vi "Resource Editor.vi"(7 "Load from Initial Path (F)":bool, 10 "Initial Resources":T1, 11 "Path":path) -> (2 "Final Resources":T1)   [LabVIEW 2018]
doc: "Edits several types of LabVIEW files at a low level, including VI's.\n\nCan also be used as a dialog subVI for editing resource clusters."
uses:
  Resource Array.ctl
  Resource.ctl
  Resource Editor Internal Commands Enum.ctl
panel:
  in  "Delete":bool
  in  "Add":bool
  in  "Name":string
  in  "Type":string
  in  "ID":i32
  in  "Export":bool
  in  "Import":bool
  in  "Paste":bool
  in  "Copy":bool
  in  "XML":bool
  in  "Fix MD5":bool
  in  "File type":string
  in  "Data":string
  in  "Hex view":bool
  in  "Save":bool
  in  "Load":bool
  in  "Resources":i32(listbox)
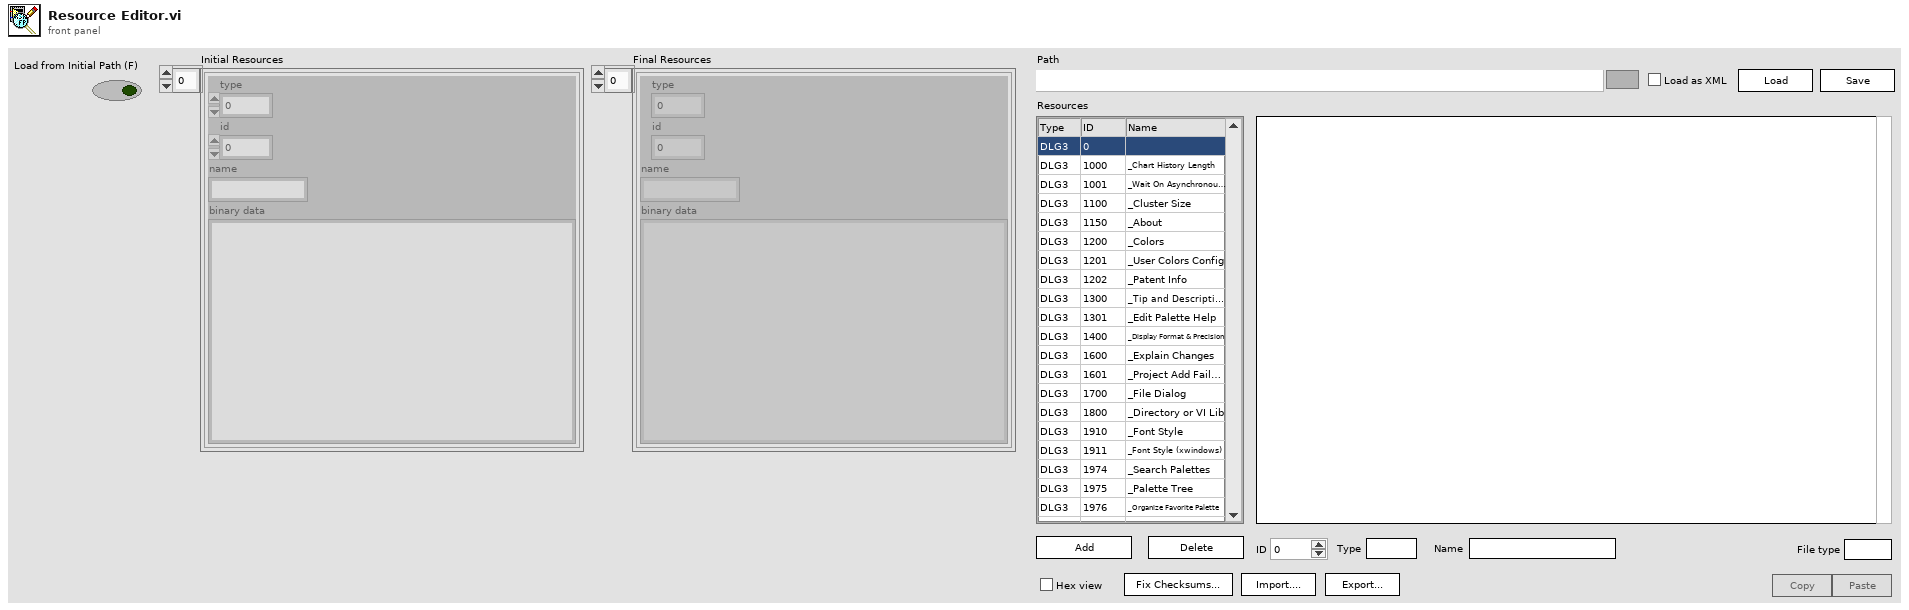
[diagram p1: front panel]
types:
  T1 = typedef "Resource Array.ctl" = T2[]
  T2 = typedef "Resource.ctl" = cluster{"type":u32, "id":i32, "name":string, "binary data":string}
  T3 = typedef "Resource Editor Internal Commands Enum.ctl" = enum16{"Refresh Resource List", "Load from Path"}
  T4 = enum8{"Enabled", "Disabled", "Disabled and Grayed Out"}
  T5 = enum16{"Left Button", "Center Button", "Right Button", "Window Close"}
  T6 = enum16{"open", "replace", "create", "open or create", "replace or create", "replace or create with confirmation"}
  T7 = cluster{"Numbers":u32, "Strings":u32, "Paths":u32}
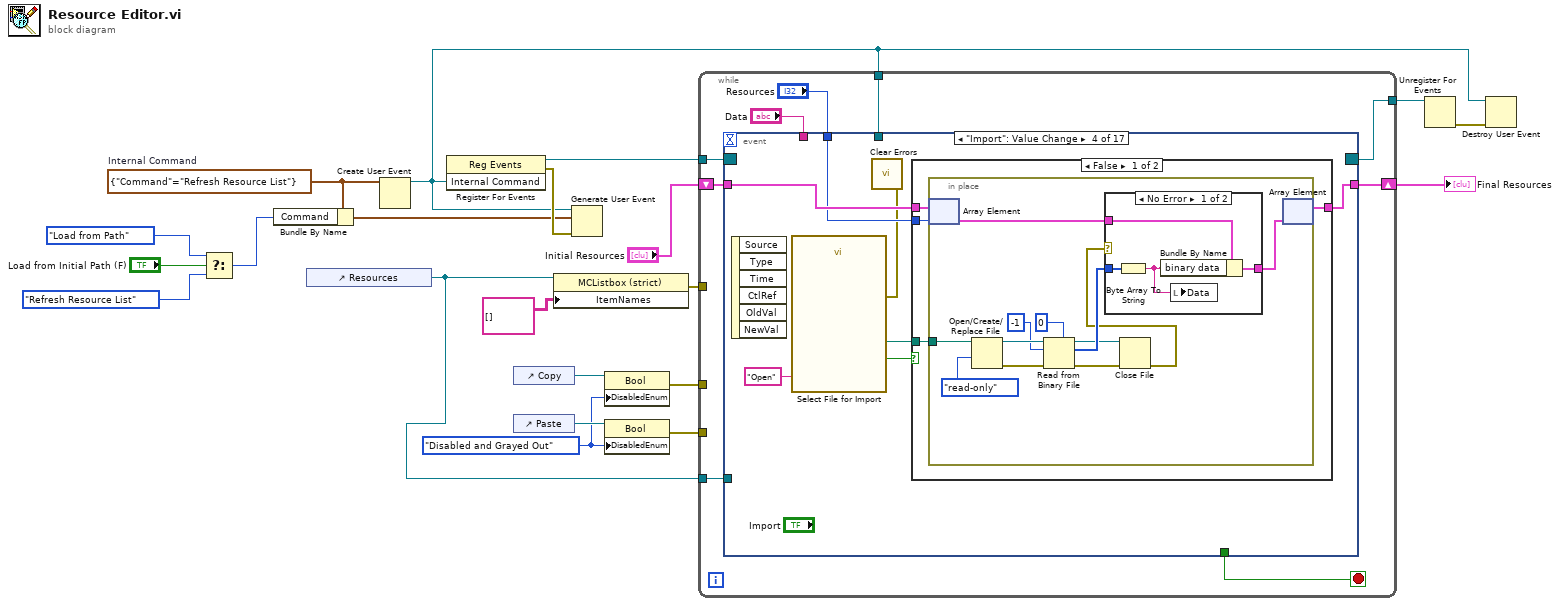
[diagram p0: block diagram]
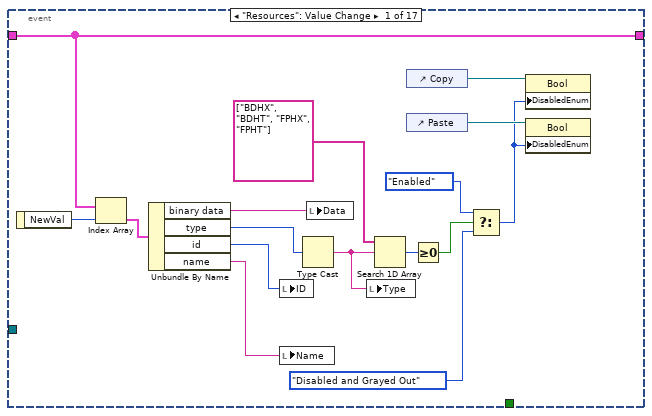
[diagram p2: hidden frame]
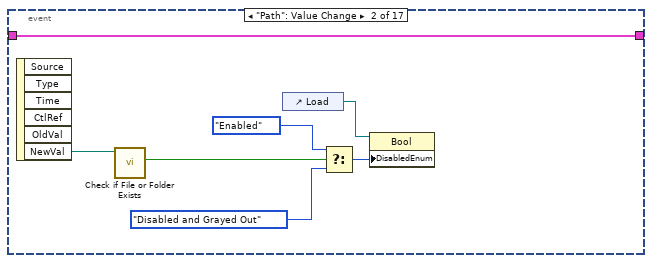
[diagram p3: hidden frame]
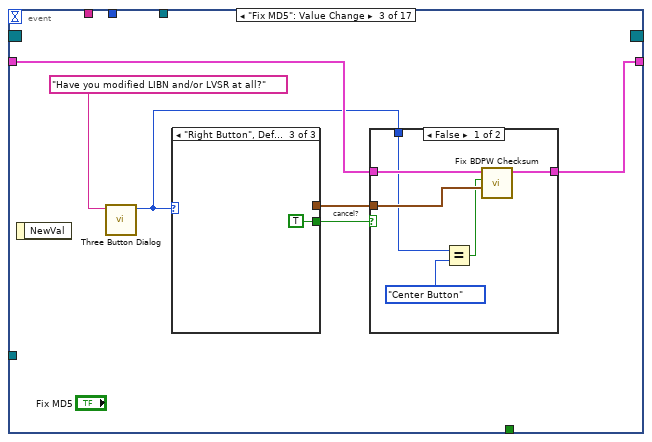
[diagram p4: hidden frame]
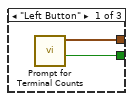
[diagram p5: hidden frame]
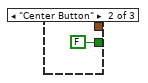
[diagram p6: hidden frame]
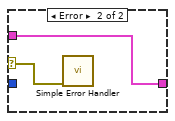
[diagram p8: hidden frame]
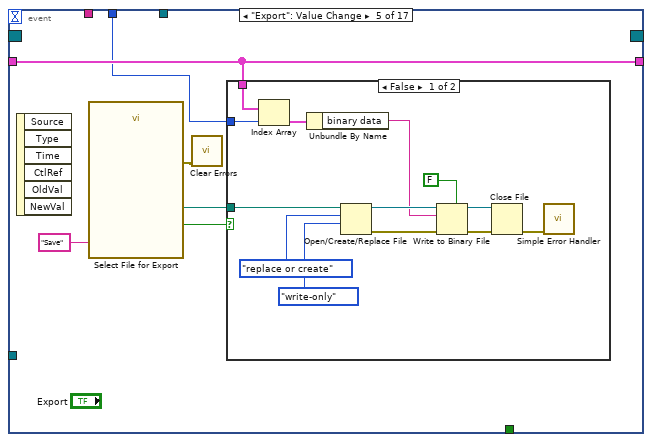
[diagram p10: hidden frame]
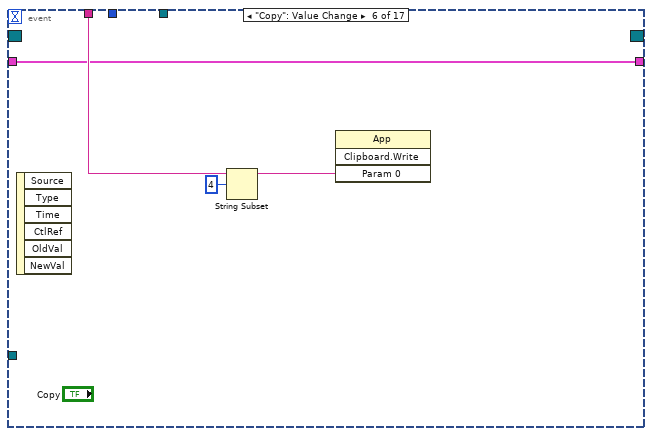
[diagram p12: hidden frame]
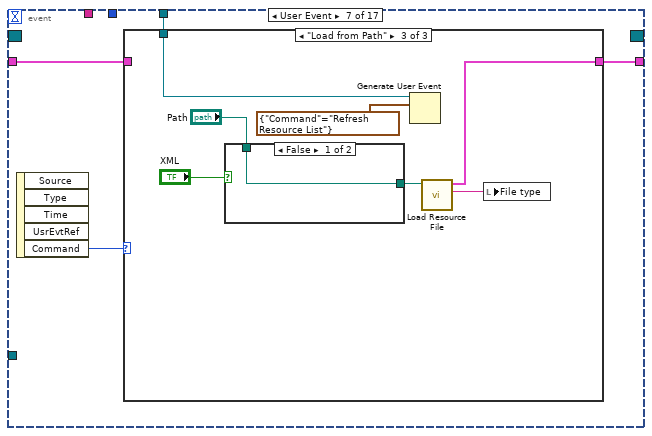
[diagram p13: hidden frame]
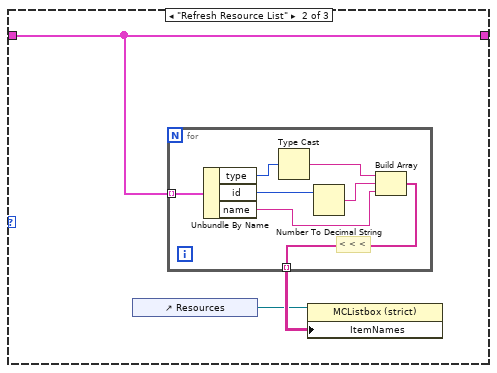
[diagram p15: hidden frame]
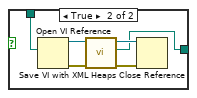
[diagram p16: hidden frame]
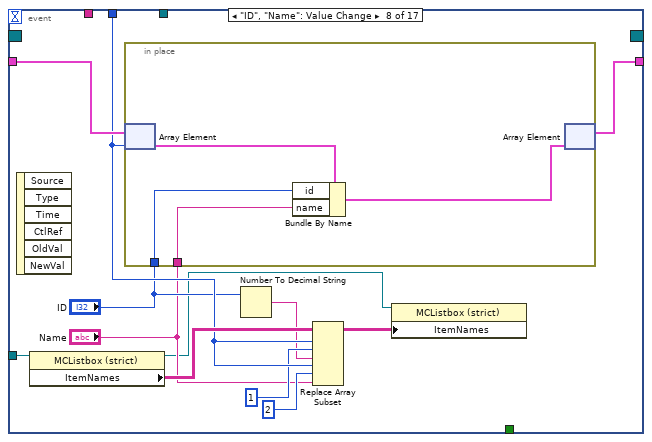
[diagram p17: hidden frame]
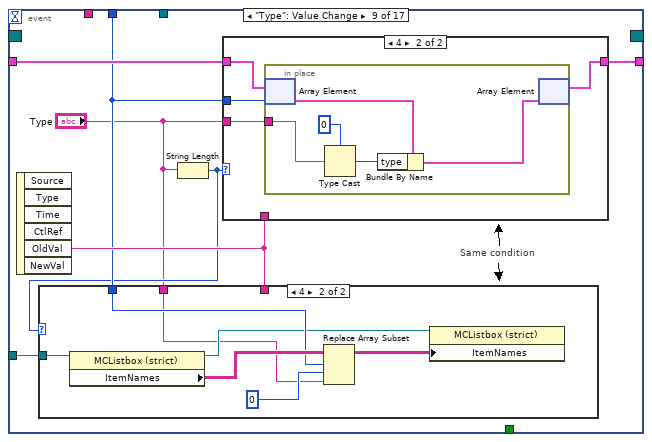
[diagram p18: hidden frame]
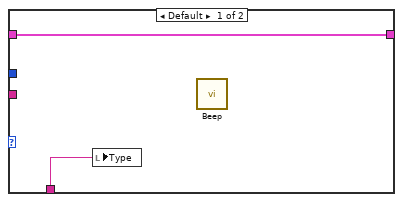
[diagram p20: hidden frame]
diagram:
  w6 = cluster{"Command":T3} {"Command"=enum."Refresh Resource List"}  # Internal Command
  w16 = T4."Disabled and Grayed Out" ("Disabled")
  n1 = Select(t=Resource_Editor_Internal_Commands_Enum."Load from Path" ("Command"), s="Load from Initial Path (F)", f=Resource_Editor_Internal_Commands_Enum."Refresh Resource List" ("Command")) -> (s? t:f=w1:T3)
  n2 = Bundle By Name(cluster=w6, "Command"=w1) -> (w5:cluster{"Command":T3})
  n3 = control-ref of="Resources"() -> (w13:refnum<vi>)
  n4 = Create User Event(user event datatype=w6) -> (user event=w7:refnum<user-event>)  [unwired: 1 in, 1 out]
  n5 = register-events(w7) -> (reference out=w8:refnum<event-registration>, error out=w9:errorcluster)  [unwired: 2 in]
  n6 = control-ref of="Copy"() -> (w18:refnum<vi>)
  n7 = control-ref of="Paste"() -> (w17:refnum<vi>)
  n8 = property class="MCListbox (strict)"(reference=w13, "ItemNames"=string[][] [] ("Item Names")) -> (error out=w20:errorcluster)  [unwired: 1 in, 1 out]
  n9 = Generate User Event(user event=w7, event data cluster=w5, error in=w9) -> ()  [unwired: 1 in, 2 out]
  n10 = property class="Bool"(reference=w18, "DisabledEnum"=w16) -> (error out=w15:errorcluster)  [unwired: 1 in, 1 out]
  n11 = property class="Bool"(reference=w17, "DisabledEnum"=w16) -> (error out=w14:errorcluster)  [unwired: 1 in, 1 out]
  n12 = while {
    shift-right: [w29] -> w12
    shift-left: "Initial Resources" -> [w30]
    tunnel: w20 -> [_]
    tunnel: w15 -> [_]
    tunnel: w14 -> [_]
    tunnel: w13 -> [w25]
    tunnel: w8 -> [w24]
    tunnel: w7 -> [w23]
    tunnel: [w22] -> w11
    stop <- w28 stop-if-true
    n13 = event shown="[3] \"Import\": Value Change" {
      selector: w24 -> [_ _ _ _ _ _ _ _ _ _ _ _ _ _ _ _ _]
      dyn-events: [_ _ _ _ _ _ _ _ _ _ _ _ _ _ _ _ _] -> w22
      timeout: _ -> [_ _ _ _ _ _ _ _ _ _ _ _ _ _ _ _ _]
      tunnel: w30 -> [w44 w47 w56 w77 w106 w122 w125 w164 w175 w202 w218 w227 w232 w239 w246 w251 w260]
      tunnel: [w44 w47 w59 w75 w106 w122 w126 w163 w174 w200 w216 w227 w232 w237 w244 w251 w260] -> w29
      tunnel: [_ _ _ _ _ _ _ _ _ _ _ _ _ _ _ _ w261] -> w28
      tunnel: "Data" -> [_ _ _ _ _ w123 _ _ _ _ _ _ _ _ _ _ _]
      tunnel: "Resources" -> [_ _ _ w76 w103 _ _ w161 w171 w201 w215 _ _ w233 w245 _ _]
      tunnel: w25 -> [_ _ _ _ _ _ _ w154 w173 _ _ _ _ _ _ _ _]
      tunnel: w23 -> [_ _ _ _ _ _ w124 _ _ _ _ _ w230 _ w243 _ _]
      event "Resources": Value Change {
        n14 = event-data() -> ("NewVal"=w46:i32)  [unwired: 1 in]
        n15 = Index Array(array=w44, index=w46) -> (element=w45:T2)
        n16 = Unbundle By Name(w45) -> ("binary data"=w43:string, "type"=w42:u32, "id"=w33:i32, "name"=w32:string)
        n17 = local write "ID"(w33) -> ()
        n18 = local write "Name"(w32) -> ()
        n19 = Type Cast(x=w42) -> (*(type *) &x=w31:string)  [unwired: 1 in]
        n20 = local write "Data"(w43) -> ()
        n21 = local write "Type"(w31) -> ()
        n22 = Search 1D Array(1D array=string[] ["BDHX", "BDHT", "FPHX", "FPHT"], element=w31) -> (index of element=w38:i32)  [unwired: 1 in]
        n23 = control-ref of="Copy"() -> (w40:refnum<vi>)
        n24 = control-ref of="Paste"() -> (w39:refnum<vi>)
        n25 = Greater Or Equal To 0?(x=w38) -> (x >= 0?=w37:bool)
        n26 = Select(t=T4."Enabled" ("Disabled"), s=w37, f=T4."Disabled and Grayed Out" ("Disabled")) -> (s? t:f=w34:T4)
        n27 = property class="Bool"(reference=w40, "DisabledEnum"=w34) -> ()  [unwired: 1 in, 2 out]
        n28 = property class="Bool"(reference=w39, "DisabledEnum"=w34) -> ()  [unwired: 1 in, 2 out]
      }
      event "Path": Value Change {
        n29 = event-data() -> ("NewVal"=w53:path)  [unwired: 1 in, 5 out]
        n30 = call <vilib>:"Check if File or Folder Exists.vi"("path"=w53) -> ("file or folder exists?"=w48:bool)  [unwired: 8 in, 2 out]
        n31 = control-ref of="Load"() -> (w52:refnum<vi>)
        n32 = Select(t=T4."Enabled" ("Disabled"), s=w48, f=T4."Disabled and Grayed Out" ("Disabled")) -> (s? t:f=w49:T4)
        n33 = property class="Bool"(reference=w52, "DisabledEnum"=w49) -> ()  [unwired: 1 in, 2 out]
      }
      event "Fix MD5": Value Change {
        # "cancel?"
        n34 = event-data() -> ()  [unwired: 1 in, 1 out]
        n35 = call <vilib>:"Three Button Dialog.vi"("message"="Have you modified LIBN and/or LVSR at all?") -> ("Which Button?"=w54:T5)  [unwired: 10 in]
        n36 = case shown="\"Right Button\", Default" w54 {
          tunnel: [w61 FALSE ("Canceled?") TRUE ("Canceled?")] -> w58
          tunnel: [w60 _ _] -> w57
          frame "Left Button" {
            n37 = call "Prompt for Terminal Counts.vi"() -> ("Canceled?"=w61:bool, "Terminal Counts"=w60:T7)  [unwired: 10 in]
          }
          frame "Center Button" {
          }
          frame "Right Button", Default {
          }
        }
        n38 = case shown="False" w58 {
          tunnel: w56 -> [w69 w70]
          tunnel: [w68 w70] -> w59
          tunnel: w57 -> [w67 _]
          tunnel: w54 -> [w65 _]
          frame False {
            n39 = Equal?(x=w65, y=T5."Center Button" ("Which Button?")) -> (x = y?=w64:bool)
            n40 = call "Fix BDPW Checksum.vi"("Terminal Counts"=w67, "Only fix 3rd hash (F)"=w64, "Resources in"=w69) -> ("Resources out"=w68:T1)  [unwired: 8 in]
          }
          frame True {
          }
        }
      }
      event "Import": Value Change {
        n41 = event-data() -> ()  [unwired: 1 in, 6 out]
        n42 = call "Select File for Import"("button label"="Open") -> ("selected path"=w73:path, "cancelled"=w74:bool, "error out"=w71:errorcluster)  [unwired: 11 in, 1 out]
        n43 = call <vilib>:"Clear Errors.vi"("error in (no error)"=w71) -> ()  [unwired: 5 in, 2 out]
        n44 = case shown="False" w74 {
          tunnel: w77 -> [w81 w100]
          tunnel: w76 -> [w80 _]
          tunnel: [w79 w100] -> w75
          tunnel: w73 -> [w78 _]
          frame False {
            n45 = in-place {
              in-place-border: w78 -> [w93]
              n46 = in-place-array #1(w81, w80) -> (w87:T2)
              n47 = Open/Create/Replace File(file path (use dialog)=w93, access (0:read/write)=enum16{"read/write", "read-only", "write-only"}."read-only") -> (refnum out=w91:refnum<file>, error out=w88:errorcluster)  [unwired: 4 in, 1 out]
              n48 = Read from Binary File(5:u8 0, 8:w88, 10:-1 ("count (1)"), 11:w91) -> (0:w83:errorcluster, 2:w86:u8[], 3:w84:refnum<file>)  [unwired: 2 in, 1 out]
              n49 = Close File(refnum=w84, error in=w83) -> (error out=w82:errorcluster)  [unwired: 1 out]
              n50 = case shown="No Error" w82 {
                selector: w82 -> [_ w98]
                tunnel: w87 -> [w97 w99]
                tunnel: w86 -> [w96 _]
                tunnel: [w95 w99] -> w85
                frame No Error {
                  n51 = Byte Array To String(unsigned byte array=w96) -> (string=w94:string)
                  n52 = Bundle By Name(cluster=w97, "binary data"=w94) -> (w95:T2)
                  n53 = local write "Data"(w94) -> ()
                }
                frame Error {
                  n54 = call <vilib>:"Simple Error Handler.vi"("error in (no error)"=w98) -> ()  [unwired: 4 in, 5 out]
                }
              }
              n55 = in-place-array #1(w85) -> (w79:T1)  [unwired: 1 out]
            }
          }
          frame True {
          }
        }
      }
      event "Export": Value Change {
        n56 = event-data() -> ()  [unwired: 1 in, 6 out]
        n57 = call "Select File for Export"("button label"="Save") -> ("selected path"=w104:path, "cancelled"=w105:bool, "error out"=w101:errorcluster)  [unwired: 11 in, 1 out]
        n58 = call <vilib>:"Clear Errors.vi"("error in (no error)"=w101) -> ()  [unwired: 5 in, 2 out]
        n59 = case shown="False" w105 {
          tunnel: w106 -> [w114 _]
          tunnel: w104 -> [w119 _]
          tunnel: w103 -> [w113 _]
          frame False {
            n60 = Index Array(array=w114, index=w113) -> (element=w112:T2)
            n61 = Unbundle By Name(w112) -> ("binary data"=w111:string)
            n62 = Open/Create/Replace File(file path (use dialog)=w119, operation (0:open)=T6."replace or create", access (0:read/write)=enum16{"read/write", "read-only", "write-only"}."write-only") -> (refnum out=w115:refnum<file>, error out=w108:errorcluster)  [unwired: 3 in, 1 out]
            n63 = Write to Binary File(file (use dialog)=w115, data=w111, error in=w108, 5:FALSE ("prepend array or string size? (T)")) -> (refnum out=w109:refnum<file>, error out=w110:errorcluster)  [unwired: 2 in, 1 out]
            n64 = Close File(refnum=w109, error in=w110) -> (error out=w107:errorcluster)  [unwired: 1 out]
            n65 = call <vilib>:"Simple Error Handler.vi"("error in (no error)"=w107) -> ()  [unwired: 4 in, 5 out]
          }
          frame True {
          }
        }
      }
      event "Copy": Value Change {
        n66 = event-data() -> ()  [unwired: 1 in, 6 out]
        n67 = String Subset(string=w123, offset (0)=4) -> (substring=w121:string)  [unwired: 1 in]
        n68 = invoke class="App" method="Clipboard.Write"("Param 0"=w121) -> ()  [unwired: 3 in, 4 out]
      }
      event User Event {
        n69 = event-data() -> ("Command"=w127:T3)  [unwired: 1 in, 4 out]
        n70 = case shown="\"Load from Path\"" w127 {
          tunnel: [w128 w130 w141] -> w126
          tunnel: w125 -> [w128 w130 _]
          tunnel: w124 -> [_ _ w139]
          frame Default {
          }
          frame "Refresh Resource List" {
            n71 = control-ref of="Resources"() -> (w129:refnum<vi>)
            n72 = for {
              tunnel: [w138] -> w131 mode=indexing
              tunnel: w130 -> [w134] mode=indexing
              # "< < <"
              n73 = Unbundle By Name(w134) -> ("type"=w137:u32, "id"=w133:i32, "name"=w132:string)
              n74 = Type Cast(x=w137) -> (*(type *) &x=w135:string)  [unwired: 1 in]
              n75 = Number To Decimal String(number=w133) -> (decimal integer string=w136:string)  [unwired: 1 in]
              n76 = Build Array(w135, w136, w132) -> (w138:string[])
            }
            n77 = property class="MCListbox (strict)"(reference=w129, "ItemNames"=w131) -> ()  [unwired: 1 in, 2 out]
          }
          frame "Load from Path" {
            n78 = case shown="False" "XML" {
              tunnel: "Path" -> [w146 w152]
              tunnel: [w146 w147] -> w144
              frame False {
              }
              frame True {
                n79 = Open VI Reference(vi path=w152) -> (vi reference=w151:refnum<vi>, error out=w150:errorcluster)  [unwired: 5 in]
                n80 = call "Save VI with XML Heaps.vi"("error in (no error)"=w150, "VI Refnum In"=w151) -> ("error out"=w149:errorcluster, "VI Path out"=w147:path, "VI Refnum Out"=w148:refnum<vi>)  [unwired: 7 in]
                n81 = Close Reference(reference=w148, error in (no error)=w149) -> ()  [unwired: 1 out]
              }
            }
            n82 = Generate User Event(user event=w139, event data cluster=cluster{"Command":T3} {"Command"=enum."Refresh Resource List"} ("event data")) -> ()  [unwired: 2 in, 2 out]
            n83 = call "Load Resource File.vi"("Resource file"=w144) -> ("File Type"=w140:string, "Resources"=w141:T1)  [unwired: 8 in, 1 out]
            n84 = local write "File type"(w140) -> ()
          }
        }
      }
      event "ID", "Name": Value Change {
        n85 = event-data() -> ()  [unwired: 1 in, 6 out]
        n86 = property class="MCListbox (strict)"(reference=w154) -> (reference out=w153:refnum<vi>, "ItemNames"=w162:string[][])  [unwired: 1 in, 1 out]
        n87 = in-place {
          in-place-border: "ID" -> [w166]
          in-place-border: "Name" -> [w165]
          n88 = in-place-array #2(w164, w161) -> (w168:T2)
          n89 = Bundle By Name(cluster=w168, "id"=w166, "name"=w165) -> (w167:T2)
          n90 = in-place-array #2(w167) -> (w163:T1)  [unwired: 1 out]
        }
        n91 = Number To Decimal String(number="ID") -> (decimal integer string=w157:string)  [unwired: 1 in]
        n92 = Replace Array Subset(array=w162, new element #1=w157, index (row) #1=w161, index (col) #1=1, new element #2="Name", index (row) #2=w161, index (col) #2=2) -> (w155:string[][])
        n93 = property class="MCListbox (strict)"(reference=w153, "ItemNames"=w155) -> ()  [unwired: 1 in, 2 out]
      }
      event "Type": Value Change {
        # "Same condition"
        n94 = event-data() -> ("OldVal"=w172:string)  [unwired: 1 in, 5 out]
        n95 = String Length(string="Type") -> (length=w170:i32)
        n96 = case shown="4" w170 {
          tunnel: w173 -> [_ w182]
          tunnel: w172 -> [_ _]
          tunnel: w171 -> [_ w180]
          tunnel: "Type" -> [_ w176]
          frame Default {
          }
          frame 4 {
            n97 = property class="MCListbox (strict)"(reference=w182) -> (reference out=w177:refnum<vi>, "ItemNames"=w181:string[][])  [unwired: 1 in, 1 out]
            n98 = Replace Array Subset(array=w181, new element=w176, index (row)=w180, index (col)=0) -> (w178:string[][])
            n99 = property class="MCListbox (strict)"(reference=w177, "ItemNames"=w178) -> ()  [unwired: 1 in, 2 out]
          }
        }
        n100 = case shown="4" w170 {
          tunnel: "Type" -> [_ w186]
          tunnel: w175 -> [w184 w188]
          tunnel: w171 -> [_ w187]
          tunnel: [w184 w185] -> w174
          tunnel: w172 -> [w183 _]
          frame Default {
            n101 = local write "Type"(w183) -> ()
            n102 = call <vilib>:"Beep.vi"() -> ()  [unwired: 12 in]
          }
          frame 4 {
            n103 = in-place {
              in-place-border: w186 -> [w192]
              n104 = in-place-array #3(w188, w187) -> (w193:T2)
              n105 = Type Cast(type=u32 0, x=w192) -> (*(type *) &x=w190:u32)
              n106 = Bundle By Name(cluster=w193, "type"=w190) -> (w189:T2)
              n107 = in-place-array #3(w189) -> (w185:T1)  [unwired: 1 out]
            }
          }
        }
      }
      event "Paste": Value Change {
        # "< < <"
        n108 = event-data() -> ()  [unwired: 1 in, 6 out]
        n109 = invoke class="App" method="Clipboard.Read"() -> (error out=w203:errorcluster, "Read Clipbrd"=w195:string)  [unwired: 3 in, 1 out]
        n110 = call "Is Big Endian.vi"() -> ("big endian"=w199:bool)
        n111 = String Length(string=w195) -> (length=w197:i32)
        n112 = Type Cast(x=w197) -> (*(type *) &x=w198:string)  [unwired: 1 in]
        n113 = case shown="True" w199 {
          tunnel: w198 -> [w204 w206]
          tunnel: [w204 w205] -> w194
          frame False {
          }
          frame True {
            n114 = Reverse String(1:w206) -> (0:w205:string)
          }
        }
        n115 = Concatenate Strings(w194, w195) -> (w196:string)
        n116 = case shown="No Error" w203 {
          tunnel: w196 -> [w208 _]
          tunnel: w202 -> [w209 w214]
          tunnel: w201 -> [w210 _]
          tunnel: [w207 w214] -> w200
          frame No Error {
            n117 = in-place {
              in-place-border: w208 -> [w211]
              n118 = in-place-array #4(w209, w210) -> (w212:T2)
              n119 = local write "Data"(w211) -> ()
              n120 = Bundle By Name(cluster=w212, "binary data"=w211) -> (w213:T2)
              n121 = in-place-array #4(w213) -> (w207:T1)  [unwired: 1 out]
            }
          }
          frame Error {
          }
        }
      }
      event "Data": Value Change {
        n122 = event-data() -> ("NewVal"=w217:string)  [unwired: 1 in]
        n123 = in-place {
          in-place-border: w217 -> [w220]
          n124 = in-place-array #5(w218, w215) -> (w221:T2)
          n125 = Bundle By Name(cluster=w221, "binary data"=w220) -> (w219:T2)
          n126 = in-place-array #5(w219) -> (w216:T1)  [unwired: 1 out]
        }
      }
      event "Hex view": Value Change {
        n127 = event-data() -> ()  [unwired: 1 in, 1 out]
        n128 = Select(t=u32 3 ("Display Style"), s="Hex view", f=u32 0 ("Display Style")) -> (s? t:f=w223:u32)
        n129 = control-ref of="Data"() -> (w226:refnum<vi>)
        n130 = property class="Str"(reference=w226, "Display Style"=w223) -> ()  [unwired: 1 in, 2 out]
      }
      event "Load": Value Change {
        n131 = event-data() -> ()  [unwired: 1 in, 1 out]
        n132 = control-ref of="Resources"() -> (w229:refnum<vi>)
        n133 = Generate User Event(user event=w230, event data cluster=cluster{"Command":T3} {"Command"=enum."Load from Path"}) -> ()  [unwired: 2 in, 2 out]
        n134 = property class="MCListbox (strict)"(reference=w229, "Val(Sgnl)"=0 ("Value (Signaling)")) -> ()  [unwired: 1 in, 2 out]
      }
      event "Add": Value Change {
        n135 = event-data() -> ()  [unwired: 1 in, 6 out]
        n136 = control-ref of="Resources"() -> (w241:refnum<vi>)
        n137 = Insert Into Array(array=w239, index=w233, new element=T2 {"type"=1315272530, "id"=0, "name"="", "binary data"=""} ("element")) -> (w237:T1)
        n138 = property class="MCListbox (strict)"(reference=w241) -> (reference out=w240:refnum<vi>, "ItemNames"=w236:string[][])  [unwired: 1 in, 1 out]
        n139 = Insert Into Array(array=w236, index (row)=w233, new element=string[] ["NewR", "0", ""]) -> (w235:string[][])  [unwired: 1 in]
        n140 = property class="MCListbox (strict)"(reference=w240, "ItemNames"=w235, "Val(Sgnl)"=w233) -> ()  [unwired: 1 in, 2 out]
      }
      event "Delete": Value Change {
        n141 = event-data() -> ()  [unwired: 1 in, 6 out]
        n142 = Delete From Array(array=w246, index=w245) -> (array with subset deleted=w244:T1)  [unwired: 1 in, 1 out]
        n143 = Generate User Event(user event=w243, event data cluster=cluster{"Command":T3} {"Command"=enum."Refresh Resource List"} ("event data")) -> ()  [unwired: 2 in, 2 out]
      }
      event "Save": Value Change {
        n144 = event-data() -> ()  [unwired: 1 in, 1 out]
        n145 = local read "Path"() -> (w247:path)
        n146 = call <vilib>:"Check if File or Folder Exists.vi"("path"=w247) -> ("file or folder exists?"=w250:bool, "dup path"=w248:path)  [unwired: 8 in, 1 out]
        n147 = case shown="False" w250 {
          tunnel: [TRUE ("T button?") w257] -> w249
          frame False {
          }
          frame True {
            n148 = Two Button Dialog(message="This file already exists. Overwrite it?", 1:"No", 2:"Yes" ("T button name (\"OK\")")) -> (T button?=w257:bool)
          }
        }
        n149 = case shown="True" w249 {
          tunnel: w251 -> [_ w254]
          tunnel: w248 -> [_ w252]
          frame False {
          }
          frame True {
            n150 = call "Save Resource File.vi"("Path"=w252, "File type"="File type", "Resources"=w254) -> ()  [unwired: 8 in, 1 out]
          }
        }
      }
      event Panel Close? {
        w261 = TRUE ("Discard?")
        n151 = event-data() -> ()  [unwired: 1 in, 1 out]
        n152 = event-data("Discard?"=w261) -> ()  [unwired: 1 in, 1 out]
      }
    }
  }
  "Final Resources" <- w12
  n153 = Unregister For Events(event registration refnum=w11) -> (error out=w10:errorcluster)  [unwired: 1 in]
  n154 = Destroy User Event(user event=w7, error in=w10) -> ()  [unwired: 1 out]
